vi "Measurement Logic.vi"(8 "error in":errorcluster, 9 "measurement configuration":T2={"FGEN Resource Name"="", "Scripts"=["", ""], "Script Names"=[], "Waveforms"=[], "Selected Script"="", "Script Trigger Settings"=""}, 10 "measure call context in":refnum<class "Measure Call Context.lvclass">) -> (0 "error out":errorcluster, 1 "measurement results":T1, 2 "measure call context out":refnum<class "Measure Call Context.lvclass">)   [LabVIEW 2025, in "Fgen Script Mode.lvclass"]
doc: "Contains the core logic for executing the measurement."
uses:
  Fgen Script Mode.lvclass
  <vilib>/Plug-In SDKs/Measurements/Measure Call Context/Measure Call Context.lvclass
  Fgen Script Mode.lvclass/Fgen Script Mode.ctl
  Measurement Results.ctl
  <vilib>/Plug-In SDKs/Clients/Session Management V1/Session Reservation/Session Reservation.lvclass
  <vilib>/Plug-In SDKs/Sessions/niFGEN/NI Session Management niFGEN.lvlib
  <vilib>/Plug-In SDKs/Sessions/niFGEN/Initialize Sessions - 1Sess.vi
  <vilib>/Plug-In SDKs/Measurements/Measure Call Context/Reserve Sessions - 1Pin.vi
  <vilib>/regexp/Match Regular Expression.xnode
  Measurement Configuration.ctl
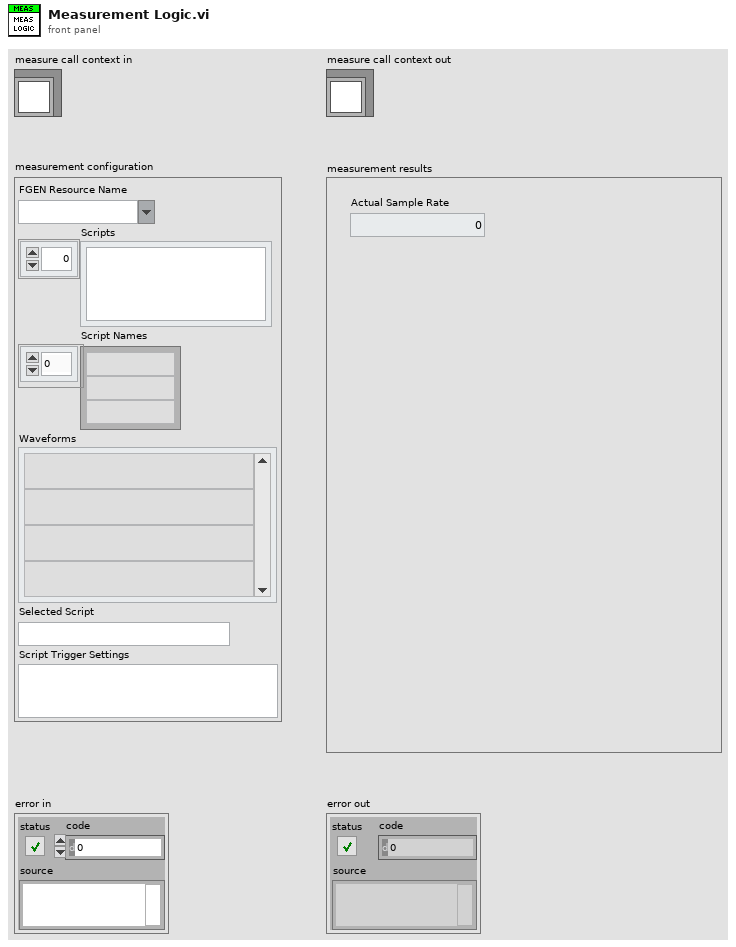
[diagram p1: front panel]
types:
  T1 = typedef "Fgen Script Mode.lvclass/Measurement Results.ctl" = cluster{"Actual Sample Rate":dbl}
  T2 = typedef "Fgen Script Mode.lvclass/Measurement Configuration.ctl" = cluster{"FGEN Resource Name":string, "Scripts":string[], "Script Names":string[], "Waveforms":string[], "Selected Script":string, "Script Trigger Settings":string}
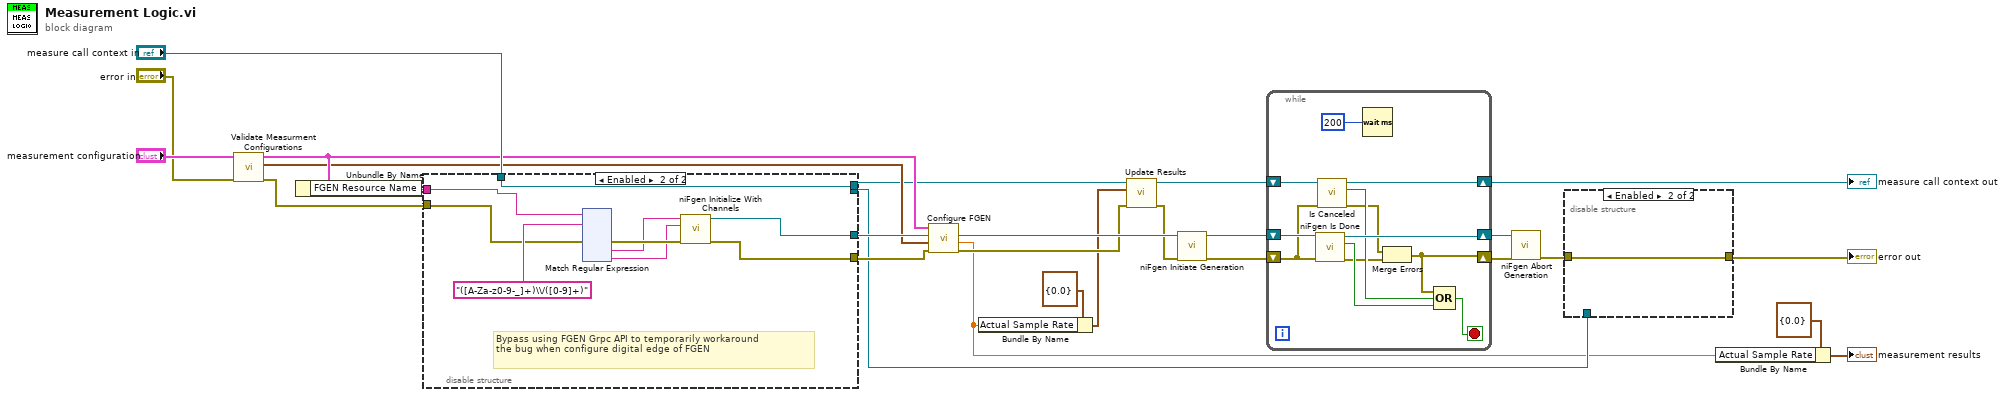
[diagram p0: block diagram]
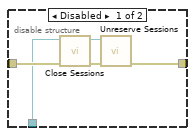
[diagram p2: hidden frame]
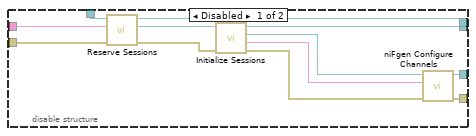
[diagram p3: hidden frame]
diagram:
  n1 = call "Validate Measurment Configurations.vi"("error in"="error in", "measurement configuration in"="measurement configuration") -> ("error out"=w2:errorcluster, "Waveforms"=w16:waveform(dbl)[], "measurement configuration out"=w18:T2)  [unwired: 7 in]
  n2 = Unbundle By Name(w18) -> ("FGEN Resource Name"=w20:string)
  n3 = disable-structure shown="Enabled" {
    disable-tunnel: "measure call context in" -> [w39 w48]
    disable-tunnel: w20 -> [w38 w46]
    disable-tunnel: [w35 w41] -> w19
    disable-tunnel: [w34 w40] -> w17
    disable-tunnel: [w31 _] -> w10
    disable-tunnel: [w30 w48] -> w7
    disable-tunnel: w2 -> [w29 w45]
    frame Disabled {
      n4 = call-poly <vilib>:"Reserve Sessions.vi"("error in"=w29, "pin or relay name"=w38, "measurement context in"=w39) -> ("error out"=w32:errorcluster, "session reservation out"=w37:refnum<class "Session Reservation.lvclass">, "measurement context out"=w30:refnum<class "Measure Call Context.lvclass">)  [unwired: 6 in]
      n5 = call-poly <vilib>:"Initialize Sessions.vi"("error in"=w32, "session reservation in"=w37) -> ("error out"=w33:errorcluster, "channel list"=w28:string, "session"=w36:refnum<k15>, "session reservation out"=w31:refnum<class "Session Reservation.lvclass">)  [unwired: 6 in]
      n6 = call <instrlib>:"niFgen Configure Channels.vi"("error in (no error)"=w33, "Channels"=w28, "Instrument Handle"=w36) -> ("error out"=w34:errorcluster, "Instrument Handle Out"=w35:refnum<k15>)  [unwired: 7 in]
    }
    frame Enabled {
      # "Bypass using FGEN Grpc API to temporarily workaround\nthe bug when configure digital edge of FGEN"
      n7 = xnode "Match Regular Expression"("input string"=w46, "regular expression"="([A-Za-z0-9-_]+)\\/([0-9]+)", "error in"=w45) -> ("error out"=w44:errorcluster, "submatch 1"=w43:string, "submatch 2"=w42:string)  [unwired: 3 in, 4 out]
      n8 = call <instrlib>:"niFgen Initialize With Channels.vi"("error in (no error)"=w44, "Channel Name"=w42, "Resource Name"=w43) -> ("error out"=w40:errorcluster, "Instrument Handle Out"=w41:refnum<k15>)  [unwired: 7 in]
    }
  }
  n9 = call "Configure FGEN.vi"("error in"=w17, "Waveforms"=w16, "FGEN Session"=w19, "measurement configuration in"=w18) -> ("error out"=w14:errorcluster, "Actual Sample Rate"=w4:dbl, "FGEN Session Out"=w15:refnum<k15>)  [unwired: 4 in, 1 out]
  n10 = Bundle By Name(cluster=T1 {"Actual Sample Rate"=0.0} ("Measurement Results"), "Actual Sample Rate"=w4) -> (w6:T1)
  n11 = call <vilib>:"Update Results.vi"("error in"=w14, "measurement results"=w6, "measure call context in"=w7) -> ("error out"=w3:errorcluster, "measure call context out"=w8:refnum<class "Measure Call Context.lvclass">)  [unwired: 7 in]
  n12 = call <instrlib>:"niFgen Initiate Generation.vi"("error in (no error)"=w3, "Instrument Handle"=w15) -> ("error out"=w1:errorcluster, "Instrument Handle Out"=w9:refnum<k15>)  [unwired: 8 in]
  n13 = while {
    shift-right: [w170] -> w13
    shift-left: w1 -> [w178]
    shift-right: [w179] -> w12
    shift-left: w9 -> [w180]
    shift-right: [w175] -> w22
    shift-left: w8 -> [w177]
    stop <- w172 stop-if-true
    n14 = call <instrlib>:"niFgen Is Done.vi"("error in (no error)"=w178, "Instrument Handle"=w180) -> ("error out"=w171:errorcluster, "Done"=w173:bool, "Instrument Handle Out"=w179:refnum<k15>)  [unwired: 7 in]
    n15 = call <vilib>:"Is Canceled.vi"("error in"=w178, "measure call context in"=w177) -> ("error out"=w169:errorcluster, "is canceled?"=w174:bool, "measure call context out"=w175:refnum<class "Measure Call Context.lvclass">)  [unwired: 7 in]
    n16 = Wait (ms)(milliseconds to wait=u32 200) -> ()  [unwired: 1 out]
    n17 = Merge Errors(w169, w171) -> (w170:errorcluster)
    n18 = Compound Arithmetic op=OR(w170, w174, w173) -> (w172:bool)
  }
  "measure call context out" <- w22
  n19 = call <instrlib>:"niFgen Abort Generation.vi"("error in (no error)"=w13, "Instrument Handle"=w12) -> ("error out"=w11:errorcluster)  [unwired: 8 in, 1 out]
  n20 = disable-structure shown="Enabled" {
    disable-tunnel: [w185 w186] -> w24
    disable-tunnel: w11 -> [w184 w186]
    disable-tunnel: w10 -> [w183 _]
    frame Disabled {
      n21 = call <vilib>:"Close Sessions.vi"("error in"=w184, "session reservation in"=w183) -> ("error out"=w182:errorcluster, "session reservation out"=w181:refnum<class "Session Reservation.lvclass">)  [unwired: 8 in]
      n22 = call <vilib>:"Unreserve Sessions.vi"("error in"=w182, "session reservation in"=w181) -> ("error out"=w185:errorcluster)  [unwired: 9 in]
    }
    frame Enabled {
    }
  }
  "error out" <- w24
  n23 = Bundle By Name(cluster=T1 {"Actual Sample Rate"=0.0} ("Measurement Results"), "Actual Sample Rate"=w4) -> (→"measurement results":T1)
